vi "Create Conditions Table.vi"(9 "HTML Options":string, 10 "Menu Items":string[](array[string]), 11 "Conditions":T1[](array[typedef])) -> (1 "HTML Conditions":string, 2 "HTML Init Values":string, 3 "Conditions Array":string[][](array[string]))   [LabVIEW 2011]
uses:
  DataFinder/DataFinder Comparisons.ctl
  DataFinder/eSearch Types.ctl
  DataFinder/Datafinder Query.ctl
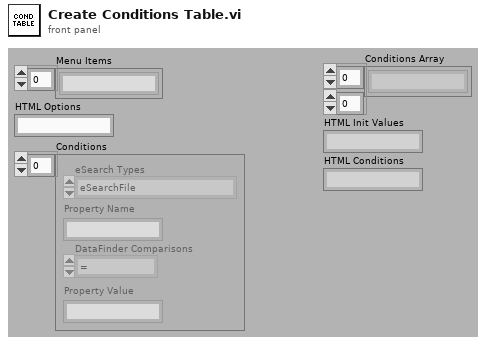
[diagram p1: front panel]
types:
  T1 = typedef "Datafinder Query.ctl" = cluster{"eSearch Types":T2, "Property Name":string, "DataFinder Comparisons":T3, "Property Value":string}
  T2 = typedef "eSearch Types.ctl" = enum16{"eSearchFile", "eSearchChannelGroup", "eSearchChannel"}
  T3 = typedef "DataFinder Comparisons.ctl" = enum16{"=", "<>", "<", "<=", ">", ">="}
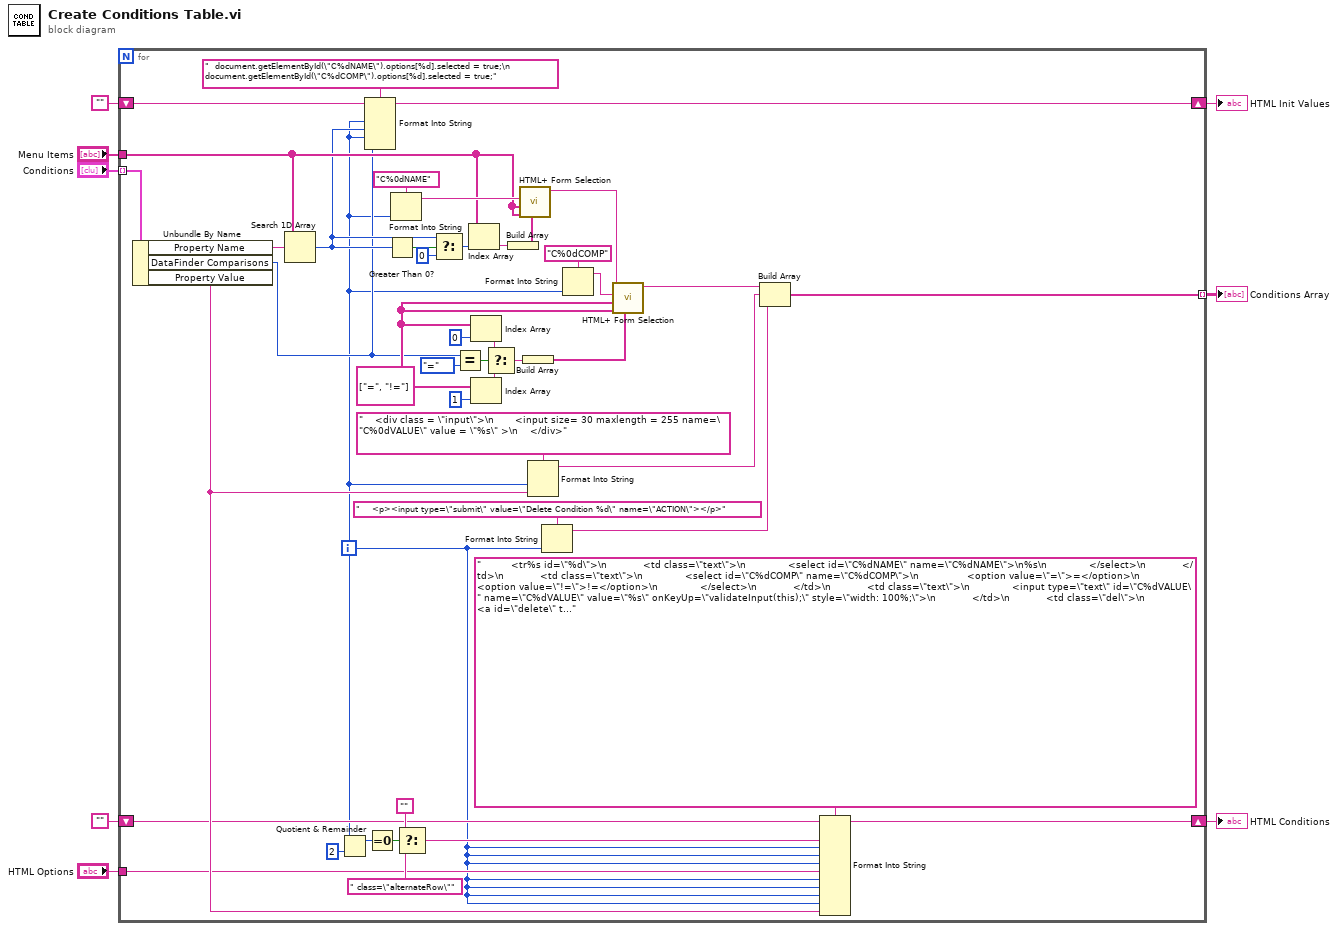
[diagram p0: block diagram]
diagram:
  n1 = for {
    tunnel: "Conditions" -> [w32] mode=indexing
    tunnel: [w37] -> w6 mode=indexing
    tunnel: "Menu Items" -> [w31]
    tunnel: "HTML Options" -> [w17]
    shift-right: [w13] -> w2
    shift-left: "" -> [w12]
    shift-right: [w11] -> w1
    shift-left: "" -> [w10]
    i -> [w9]
    w48 = string[] ["=", "!="]
    n2 = Unbundle By Name(w32) -> ("Property Name"=w38:string, "DataFinder Comparisons"=w14:T3, "Property Value"=w18:string)
    n3 = Search 1D Array(1D array=w31, element=w38) -> (index of element=w15:i32)  [unwired: 1 out]
    n4 = Quotient & Remainder(x=w9, y=2) -> (x-y*floor(x/y)=w24:i32)  [unwired: 1 out]
    n5 = Format Into String(format string="  document.getElementById(\"C%dNAME\").options[%d].selected = true;\n  document.getElementById(\"C%dCOMP\").options[%d].selected = true;" ("key"), initial string=w12, w9, w15, w9, w14) -> (resulting string=w13:string)  [unwired: 1 in, 1 out]
    n6 = Equal To 0?(x=w24) -> (x = 0?=w21:bool)
    n7 = Greater Than 0?(x=w15) -> (x > 0?=w28:bool)
    n8 = Format Into String(format string="C%0dNAME" ("key"), w9) -> (resulting string=w33:string)  [unwired: 2 in, 1 out]
    n9 = Select(t="", s=w21, f=" class=\"alternateRow\"") -> (s? t:f=w19:string)
    n10 = Select(t=w15, s=w28, f=0 ("index")) -> (s? t:f=w27:i32)
    n11 = Equal?(x=w14, y=DataFinder_Comparisons."=") -> (x = y?=w51:bool)
    n12 = Index Array(array=w31, index=w27) -> (element=w43:string)
    n13 = Index Array(array=w48, index=0) -> (element=w49:string)
    n14 = Index Array(array=w48, index=1) -> (element=w45:string)
    n15 = Select(t=w49, s=w51, f=w45) -> (s? t:f=w50:string)
    n16 = Build Array(w43) -> (w44:string[])
    n17 = call <vilib>:"HTML+ Form Selection.vi"("selected names"=w44, "item values"=w31, "item names"=w31, "name"=w33) -> ("html form content out"=w41:string)  [unwired: 3 in, 4 out]
    n18 = Build Array(w50) -> (w53:string[])
    n19 = Format Into String(format string="    <div class = \"input\">\n       <input size= 30 maxlength = 255 name=\"C%0dVALUE\" value = \"%s\" >\n    </div>", w9, w18) -> (resulting string=w39:string)  [unwired: 2 in, 1 out]
    n20 = Format Into String(format string="    <p><input type=\"submit\" value=\"Delete Condition %d\" name=\"ACTION\"></p>" ("key"), w9) -> (resulting string=w29:string)  [unwired: 2 in, 1 out]
    n21 = Format Into String(format string="C%0dCOMP" ("key"), w9) -> (resulting string=w34:string)  [unwired: 2 in, 1 out]
    n22 = call <vilib>:"HTML+ Form Selection.vi"("selected names"=w53, "item values"=w48, "item names"=w48, "name"=w34, "html form content in"=w41) -> ("html form content out"=w40:string)  [unwired: 2 in, 4 out]
    n23 = Build Array(w40, w39, w29) -> (w37:string[])
    n24 = Format Into String(format string="          <tr%s id=\"%d\">\n            <td class=\"text\">\n              <select id=\"C%dNAME\" name=\"C%dNAME\">\n%s\n              </select>\n            </td>\n            <td class=\"text\">\n              <select id=\"C%dCOMP\" name=\"C%dCOMP\">\n                <option value=\"=\">=</option>\n                <option value=\"!=\">!=</option>\n              </select>\n            </td>\n            <td class=\"text\">\n              <input type=\"text\" id=\"C%dVALUE\" name=\"C%dVALUE\" value=\"%s\" onKeyUp=\"validateInput(this);\" style=\"width: 100%;\">\n            </td>\n            <td class=\"del\">\n              <a id=\"delete\" title=\"Remove Condition\" target=\"BODY\" href=\"#nogo\" onClick=\"removeCondition(this.parentNode.parentNode.id);\"></a>\n            </td>\n          </tr>" ("key"), initial string=w10, w19, w9, w9, w9, w17, w9, w9, w9, w9, w18) -> (resulting string=w11:string)  [unwired: 1 in, 1 out]
  }
  "Conditions Array" <- w6
  "HTML Init Values" <- w2
  "HTML Conditions" <- w1
